vi "deleteEndString.vi"(8 "chars to delete":i32, 11 "string in":string) -> (3 "substring out":string)   [LabVIEW 2010]
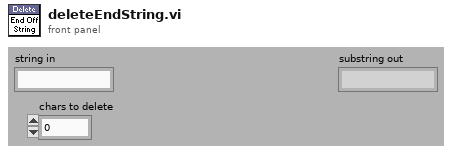
[diagram p1: front panel]
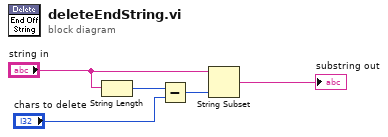
[diagram p0: block diagram]
diagram:
  n1 = String Length(string="string in") -> (length=w5:i32)
  n2 = Subtract(x=w5, y="chars to delete") -> (x-y=w4:i32)
  n3 = String Subset(string="string in", length (rest)=w4) -> (substring=→"substring out":string)  [unwired: 1 out]
